vi "FactoryCreate.vi"(8 "Error In":errorcluster, 10 "InstrumentConfig":T1, 11 "reference in":refnum<class "VdDigitalControl_Simulated.lvclass">) -> (0 "Error Out":errorcluster, 3 "reference out":refnum<class "VdDigitalControl_Simulated.lvclass">)   [LabVIEW 2020, in "VdDigitalControl_Simulated.lvclass"]
uses:
  VdDigitalControl_Simulated.lvclass
  VdInstrument_class/InstrumentConfig.ctl
  VdInstrument_class/InstrumentType.ctl
  VdDigitalControl_Simulated.lvclass/VdDigitalControl_Simulated.ctl
  VdInstrument_class/VdInstrument.lvclass
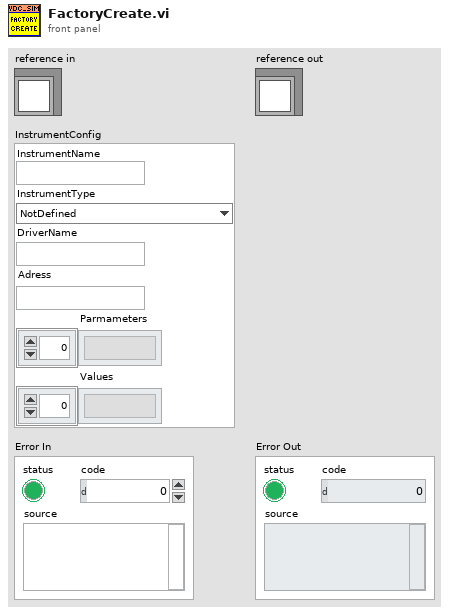
[diagram p1: front panel]
types:
  T1 = typedef "VdInstrument.lvclass/InstrumentConfig.ctl" = cluster{"InstrumentName":string, "InstrumentType":T2, "DriverName":string, "Adress":string, "Parmameters":string[], "Values":string[]}
  T2 = typedef "VdInstrument.lvclass/InstrumentType.ctl" = enum16{"NotDefined", "AirflowController", "AnalogInput", "AnalogOutput", "AutoCollimator", "BeamProfiler", "DMM", "DigitalControl", "DigitalInput", "DisplacementSensor", "Encoder", "ForceSensor", "FrequencyCounter", "FunctionGenerator", "GelDispensingRobot", "GlueDispenser", "Hexapod", "IRCamera", "ImageGenerator", "LabelPrinter", "LightController", "LightIndicator", "Load", "Multimeter", "OpticalAttenuatorPowerMeter", "OpticalChannelMonitor", "OpticalLaser", "OpticalPolarizationController", "OpticalPowerAttenuator", "OpticalPowerMeter", "OpticalSpectrumAnalyzer", "PDLMeter", "PolarisationScrambler", "PolarizationAnalyzer", "PositionSensitiveDetector", "PowerSupply", "PressureController", "Robot", "SLRCamera", "ScrewdriverController", "SignalAnalyzer", "SignalGenerator", "SixAxisStage", "SolderingStation", "SpectrumAnalyzer", "StepperMotor", "Stirrer", "SweptWavelengthSystem", "Switch", "TemperatureChamber", "TemperatureController", "TemperatureSensor", "TunableLaser", "UVCuring", "UsbHub", "VisionCamera", "WavelengthMeter", "WeldingLaser"}
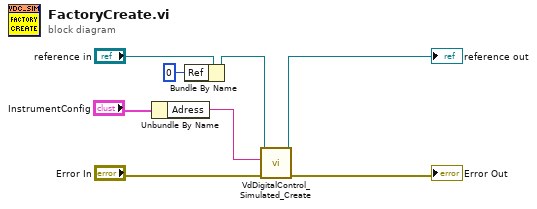
[diagram p0: block diagram]
diagram:
  n1 = Unbundle By Name("InstrumentConfig") -> ("Adress"=w1:string)
  n2 = Bundle By Name(cluster="reference in", "Ref"=u32 0) -> (w4:refnum<class "VdDigitalControl_Simulated.lvclass">)
  n3 = call "VdDigitalControl_Simulated_Create.vi"("Error In"="Error In", "Address"=w1, "reference in"=w4) -> ("Error Out"=→"Error Out":errorcluster, "reference out"=→"reference out":refnum<class "VdDigitalControl_Simulated.lvclass">)  [unwired: 7 in]
